vi "Load Glb.vi"() -> ()   [LabVIEW 2019]
panel:
  in  "Loading Exit":bool
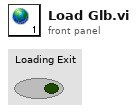
[diagram p1: front panel]
diagram:
